vi "motor_control_close_loop.vi"() -> ()   [LabVIEW 2014]
uses:
  <vilib>/platform/TimedLoop/XDataNode/XDataNode.xnode
  <vilib>/Platform/TimedLoop/XDataNode/nitl_modes.ctl
  <vilib>/Platform/TimedLoop/XDataNode/XDNodeRunTimeDep.lvlib
  <vilib>/Platform/TimedLoop/XDataNode/wakeup.ctl
  <vilib>/Platform/TimedLoop/XDataNode/timing_clust.ctl
  <vilib>/myRIO/Express VI/Onboard IO/PWM/PWM Express VI.xnode
  <vilib>/myRIO/Instrument Drivers/Onboard IO/PWM/vis/Set Duty Cycle and Frequency.vi
  <vilib>/myRIO/Instrument Drivers/Onboard IO/PWM/PWM.lvlib
  <vilib>/myRIO/Instrument Drivers/Onboard IO/PWM/typedefs/PWM Configuration.ctl
  <vilib>/myRIO/Common/Instrument Driver Framework/myRIO v1.0/PWM/typedefs/PWM Channels Enum.ctl
  <vilib>/myRIO/Common/Instrument Driver Framework/Utilities/typedefs/Generic FPGA Reference.ctl
  <vilib>/myRIO/Common/Instrument Driver Framework/Utilities/typedefs/myRIO v1.0 Reference.ctl
  <vilib>/myRIO/Common/Instrument Driver Framework/Utilities/typedefs/Hardware Version Enum.ctl
  <vilib>/myRIO/Common/Instrument Driver Framework/Utilities/typedefs/myRIO Generic Hardware Reference.ctl
  <vilib>/myRIO/Instrument Drivers/Onboard IO/PWM/typedefs/PWM Reference.ctl
  <vilib>/myRIO/Instrument Drivers/Onboard IO/PWM/vis/myRIO PWM Open.xnode
  <vilib>/myRIO/Common/Instrument Driver Framework/Utilities/vis/Is FPGA Ref Available.vi
  <vilib>/myRIO/Common/Instrument Driver Framework/myRIO v1.0/PWM/vis/myRIO v1.1 Open PWM.vi
  <vilib>/userdefined/High Color/nirio_resource_hc.ctl
  <vilib>/myRIO/Express VI/Onboard IO/Encoder/Encoder Express VI.xnode
  <vilib>/myRIO/Instrument Drivers/Onboard IO/Encoder/vis/Read.vi
  <vilib>/myRIO/Instrument Drivers/Onboard IO/Encoder/Encoder.lvlib
  <vilib>/myRIO/Common/Instrument Driver Framework/myRIO v1.0/Encoder/typedefs/Encoder Signal Mode.ctl
  <vilib>/myRIO/Common/Instrument Driver Framework/myRIO v1.0/Encoder/typedefs/Encoder Channels Enum.ctl
  <vilib>/myRIO/Instrument Drivers/Onboard IO/Encoder/typedefs/Encoder Reference.ctl
  <vilib>/myRIO/Instrument Drivers/Onboard IO/Encoder/vis/myRIO Encoder Open.xnode
  <vilib>/myRIO/Common/Instrument Driver Framework/myRIO v1.0/Encoder/vis/myRIO v1.1 Open Encoder.vi
  <vilib>/myRIO/Common/Instrument Driver Framework/myRIO v1.0/Encoder/vis/myRIO v1.0 Configure Encoder.vi
  <vilib>/myRIO/Common/Instrument Driver Framework/myRIO v1.0/Encoder/typedefs/Encoder Configuration v1.0.ctl
  <vilib>/addons/control/pid/NI_PID_pid.lvlib
  <vilib>/addons/control/pid/pid.llb/PID (DBL).vi
panel:
  out "position_B":i32
  in  "Reset_B":bool
  out "velocity_B":dbl(graph)
  out "velocity_A":dbl(graph)
  in  "Reset_A":bool
  out "position_A":i32
  in  "电机开关":bool
  in  "B_Duty":dbl(slide) scale=-1.0..1.0
  in  "关闭程序":bool
  in  "A_Duty":dbl(slide) scale=-1.0..1.0
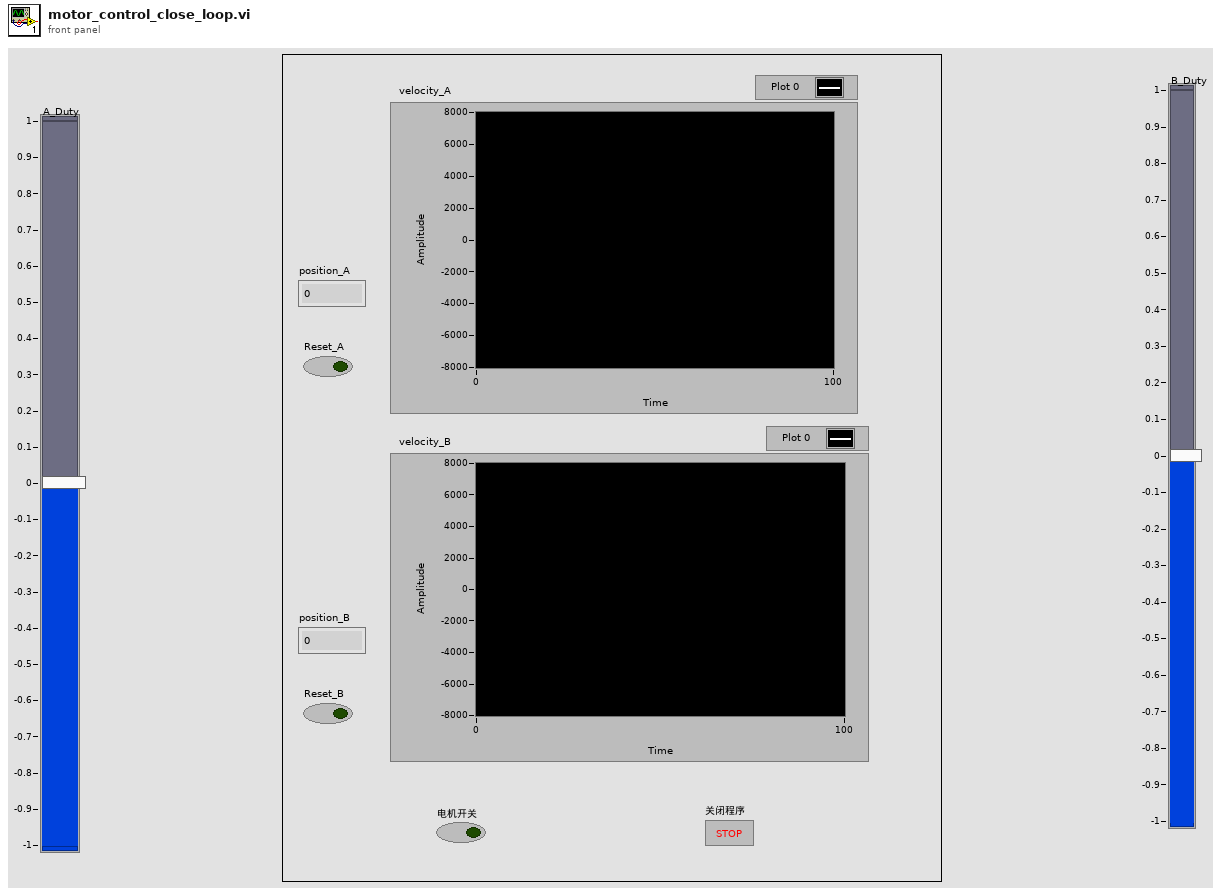
[diagram p1: front panel]
types:
  T1 = typedef "XDNodeRunTimeDep.lvlib/timing_clust.ctl" = cluster{"Expected End [f-1]":u64, "Actual End [f-1]":u64, "Finished Late? [f-1]":bool, "Expected End [i-1]":u64, "Actual End [i-1]":u64, "Finished Late? [i-1]":bool, "Expected Start [i]":u64, "Actual Start [i]":u64, "Expected Start [f]":u64, "Actual Start [f]":u64, "Source Name":string, "Structure Name":string, "Period":i64, "Deadline":i64, "Offset":i64, "Start":i64, "Priority":i32, "Timeout":i32, "Mode":T2, "Wakeup Reason":T3, "Error":errorcluster, "Source Type":string, "Secondary Source Type":string, "Global End Time":u64, "Global Start Time":u64, "Frame Duration":u64, "Iteration Duration":u64, "Assigned CPU":i32, "I/O Scan Engine Mode":u32}
  T2 = typedef "XDNodeRunTimeDep.lvlib/nitl_modes.ctl" = enum32{"No Change", "Process missed periods, maintain original phase", "Discard missed periods, maintain original phase", "Process missed periods, ignore original phase", "Discard missed periods, ignore original phase"}
  T3 = typedef "XDNodeRunTimeDep.lvlib/wakeup.ctl" = enum32{"Normal", "Aborted", "Asynchronous wakeup", "Timing source error", "Timed loop error", "Timeout"}
  T4 = typedef "Encoder.lvlib/Encoder Reference.ctl" = cluster{"myRIO Reference":T5, "Encoder Channels Enum":T9}
  T5 = typedef "myRIO Generic Hardware Reference.ctl" = cluster{"myRIO Model":T6, "myRIO Hardware Reference":T7}
  T6 = typedef "Hardware Version Enum.ctl" = enum16{"Unknown", "myRIO-1900", "myRIO-1950"}
  T7 = typedef "myRIO v1.0 Reference.ctl" = cluster{"Generic FPGA Reference":T8, "Allow multiple opens":bool}
  T8 = typedef "Generic FPGA Reference.ctl" = refnum<k20>
  T9 = typedef "Encoder Channels Enum.ctl" = enum16{"Not Connected", "C/ENC0", "C/ENC1", "A/ENC", "B/ENC"}
  T10 = typedef "Encoder Signal Mode.ctl" = enum16{"Quadrature phase signal", "Step and direction signal"}
  T11 = typedef "nirio_resource_hc.ctl" = tag
  T12 = typedef "PWM.lvlib/PWM Reference.ctl" = cluster{"myRIO Reference":T5, "PWM Channels Enum":T13, "PWM Configuration":T14}
  T13 = typedef "PWM Channels Enum.ctl" = enum16{"Not Connected", "C/PWM0", "C/PWM1", "A/PWM0", "A/PWM1", "A/PWM2", "B/PWM0", "B/PWM1", "B/PWM2"}
  T14 = typedef "PWM.lvlib/PWM Configuration.ctl" = cluster{"Frequency":dbl, "Duty Cycle":dbl}
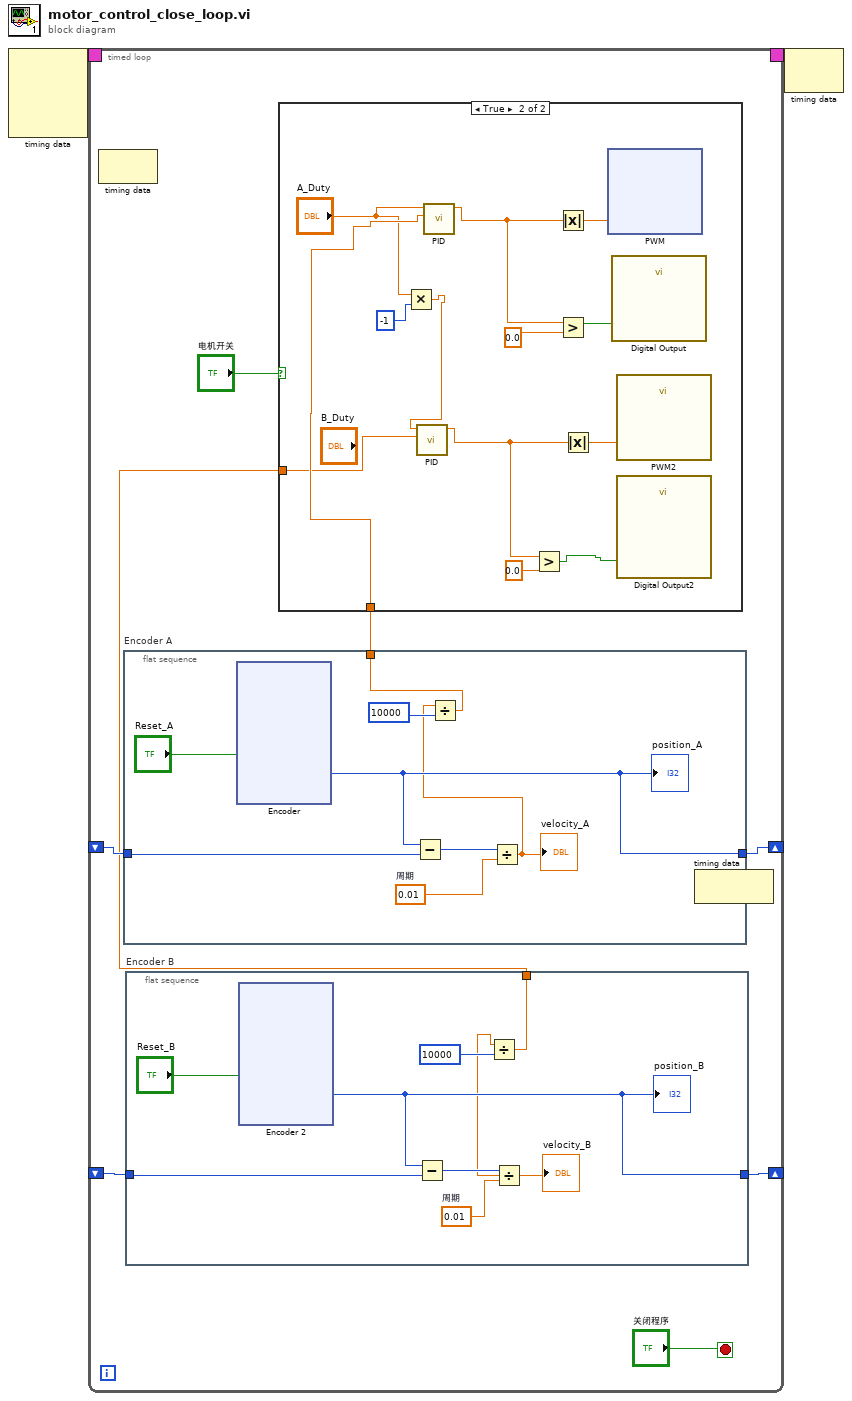
[diagram p0: block diagram]
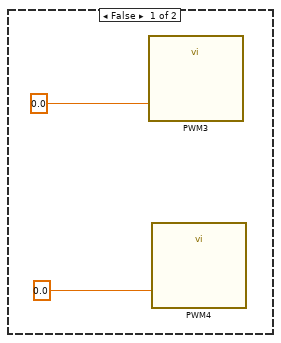
[diagram p2: hidden frame]
diagram:
  n1 = node-c288() -> (w2:T1)  [unwired: 4 in]
  n2 = timed-loop {
    timing: w2 -> [_]
    timing-out: [_] -> w1
    shift-right: [w8] -> _
    shift-left: _ -> [w7]
    shift-right: [w5] -> _
    shift-left: _ -> [w6]
    stop <- "关闭程序" stop-if-true
    n3 = node-c288() -> ()  [unwired: 1 in, 1 out]
    n4 = flat-sequence "Encoder A" {
      tunnel: [w71] -> w8
      tunnel: w7 -> [w70]
      tunnel: [w66] -> w4
      frame #0 {
        w68 = 0.01  # 周期
        n5 = xnode "Encoder"("Reset Counter"="Reset_A") -> ("Counter Value"=w71:i32)  [unwired: 1 in, 3 out]
        "position_A" <- w71
        n6 = Subtract(x=w71, y=w70) -> (x-y=w69:i32)
        n7 = Divide(x=w69, y=w68) -> (x/y=w65:dbl)
        "velocity_A" <- w65
        n8 = Divide(x=w65, y=10000) -> (x/y=w66:dbl)
      }
    }
    n9 = flat-sequence "Encoder B" {
      tunnel: [w17] -> w5
      tunnel: w6 -> [w16]
      tunnel: [w11] -> w3
      frame #0 {
        w14 = 0.01  # 周期
        n10 = xnode "Encoder 2"("Reset Counter"="Reset_B") -> ("Counter Value"=w17:i32)  [unwired: 1 in, 3 out]
        "position_B" <- w17
        n11 = Subtract(x=w17, y=w16) -> (x-y=w15:i32)
        n12 = Divide(x=w15, y=w14) -> (x/y=w12:dbl)
        "velocity_B" <- w12
        n13 = Divide(x=w12, y=10000) -> (x/y=w11:dbl)
      }
    }
    n14 = case shown="True" "电机开关" {
      tunnel: w4 -> [_ w128]
      tunnel: w3 -> [_ w126]
      frame False {
        n15 = call "PWM3"("Duty Cycle (0-1)"=0.0) -> ()  [unwired: 26 in, 1 out]
        n16 = call "PWM4"("Duty Cycle (0-1)"=0.0) -> ()  [unwired: 26 in, 1 out]
      }
      frame True {
        n17 = Multiply(x="A_Duty", y=-1) -> (x*y=w122:dbl)
        n18 = call-poly <vilib>:"PID.vi"("process variable"=w126, "setpoint"=w122) -> ("output"=w127:dbl)  [unwired: 8 in, 1 out]
        n19 = call-poly <vilib>:"PID.vi"("process variable"=w128, "setpoint"="A_Duty") -> ("output"=w129:dbl)  [unwired: 8 in, 1 out]
        n20 = Greater?(x=w127, y=0.0) -> (0:w121:bool)
        n21 = Absolute Value(x=w129) -> (abs(x)=w132:dbl)
        n22 = Greater?(x=w129, y=0.0) -> (0:w125:bool)
        n23 = Absolute Value(x=w127) -> (abs(x)=w130:dbl)
        n24 = xnode "PWM"("Duty Cycle"=w132) -> ()  [unwired: 1 in, 1 out]
        n25 = call "Digital Output"("A/DIO0 (Pin 11)"=w125) -> ()  [unwired: 26 in, 1 out]
        n26 = call "PWM2"("Duty Cycle (0-1)"=w130) -> ()  [unwired: 26 in, 1 out]
        n27 = call "Digital Output2"("B/DIO0 (Pin 11)"=w121) -> ()  [unwired: 26 in, 1 out]
      }
    }
    n28 = node-c288() -> ()  [unwired: 1 in, 1 out]
  }
  n29 = node-c288(w1) -> ()  [unwired: 1 out]
